vi "FindXMenuItem.vi"(8 "error in (no error)":errorcluster, 9 "ItemTag":string, 11 "CMenu in":refnum<class "CMenu.lvclass">) -> (0 "error out":errorcluster, 1 "Index":i32, 3 "CMenu out":refnum<class "CMenu.lvclass">)   [LabVIEW 2020, in "CMenu.lvclass"]
doc: "Search a Item.\nIf Item dose not exist, return -1, otherwise return index of item."
uses:
  CMenu.lvclass
  CMenu.lvclass/CMenu.ctl
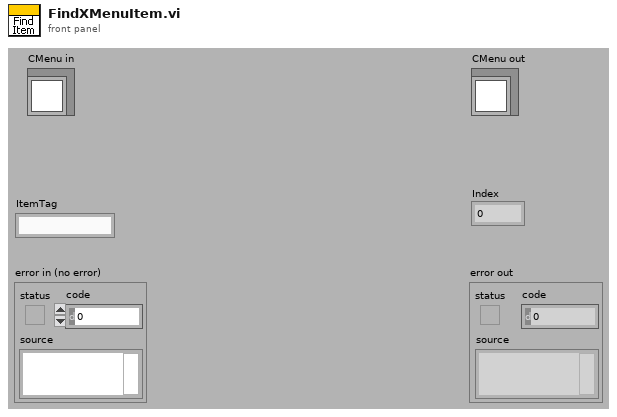
[diagram p1: front panel]
types:
  T1 = cluster{"Tag":string, "Name":string, "Symbol":i32, "Checked":bool, "ParentTag":string}[]
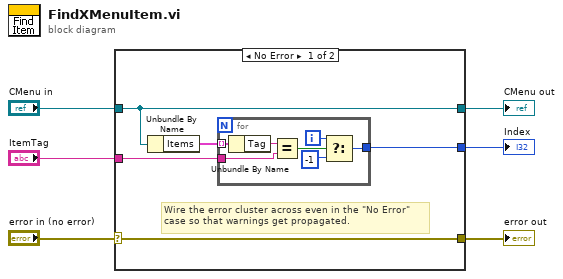
[diagram p0: block diagram]
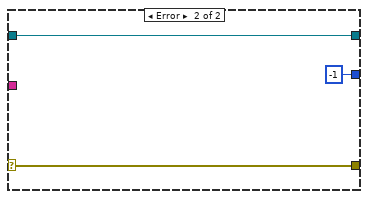
[diagram p2: hidden frame]
diagram:
  n1 = case shown="No Error" "error in (no error)" {
    selector: "error in (no error)" -> [w11 w21]
    tunnel: [w11 w21] -> w5
    tunnel: [w10 w20] -> w3
    tunnel: "CMenu in" -> [w10 w20]
    tunnel: "ItemTag" -> [w9 _]
    tunnel: [w7 -1 ("f")] -> w1
    frame No Error {
      # "Wire the error cluster across even in the \"No Error\"\ncase so that warnings get propagated."
      n2 = Unbundle By Name(w10) -> ("Items"=w8:T1)
      n3 = for {
        tunnel: w9 -> [w16]
        tunnel: w8 -> [w18] mode=indexing
        tunnel: [w12] -> w7
        i -> [w14]
        n4 = Unbundle By Name(w18) -> ("Tag"=w17:string)
        n5 = Equal?(x=w17, y=w16) -> (x = y?=w15:bool)
        n6 = Select(t=w14, s=w15, f=-1) -> (s? t:f=w12:i32)
      }
    }
    frame Error {
    }
  }
  "error out" <- w5
  "CMenu out" <- w3
  "Index" <- w1
